vi "Periodic Tasks.vi"(8 "error in":errorcluster) -> ()   [LabVIEW 2014]
doc: "This VI runs in parallel to other tasks. It can contain as many user-defined periodic loops as you need. These can carry out PID or other sorts of timed response."
uses:
  <vilib>/Rock Robotics/WPI/Joystick/WPI_JoystickGetSetRefNum.vi
  <vilib>/Rock Robotics/WPI/RobotDrive/WPI_RobotDriveGetSetRefNum.vi
  Robot Global Data.vi
  <vilib>/Rock Robotics/Network Tables/SD Write Numeric Array.vi
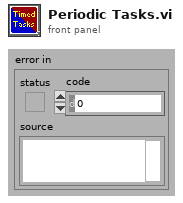
[diagram p1: front panel]
types:
  T1 = typedef "WPI_JoystickDevRef.ctl" = cluster{"Device":T2}
  T2 = typedef "WPI_JoystickDeviceEnum.ctl" = enum16{"USB 0", "USB 1", "USB 2", "USB 3", "USB 4", "USB 5"}
  T3 = typedef "WPI_RobotDriveDevRef.ctl" = cluster{"DevStatus":errorcluster, "Motors[]":T4[], "Square Inputs":bool, "Max Output":dbl}
  T4 = typedef "WPI_MotorControlDeviceRef.ctl" = cluster{"DeviceStatus":errorcluster, "Type":T5, "PWM":cluster{"Controller":T6, "PWM Channel":T7, "DeadBand":T8}, "CAN":cluster{"Device Number":u8, "Control Mode":T9, "Semaphore":T10, "Max Vout":dbl, "TalonSRX Control Mode":T11}, "Invert":bool, "TransformRef":T12, "InvTransformRef":T12}
  T5 = typedef "WPI_MotorControlType.ctl" = enum16{"PWM", "CAN", "CANTalonSRX"}
  T6 = typedef "FPGA_TypedefDigitalModule.ctl" = enum16{"Controller 1"}
  T7 = typedef "FPGA_DIOPWMChannel.ctl" = enum8{"PWM 0", "PWM 1", "PWM 2", "PWM 3", "PWM 4", "PWM 5", "PWM 6", "PWM 7", "PWM 8", "PWM 9", "PWM MXP 0", "PWM MXP 1", "PWM MXP 2", "PWM MXP 3", "PWM MXP 4", "PWM MXP 5", "PWM MXP 6", "PWM MXP 7", "PWM MXP 8", "PWM MXP 9", "Invalid"}
  T8 = typedef "WPI_PWMDeadband.ctl" = cluster{"Name":string, "maxPositivePwm":i32, "minPositivePwm":i32, "centerPwm":i32, "maxNegativePwm":i32, "minNegativePwm":i32, "angularRange":u16}
  T9 = typedef "WPI_CANJaguar_ControlMode.ctl" = enum8{"Percent VBus", "Current", "Speed", "Position", "Voltage"}
  T10 = typedef "Semaphore RefNum" = refnum<k1>
  T11 = typedef "WPI_CANTalonSRX_APIControlMode.ctl" = enum8{"Percent VBus", "Speed", "Position", "Slave", "Unchanged / Invalid"}
  T12 = typedef "WPI_PWMTransform_ConPane.ctl" = refnum<vi>
  T13 = cluster{"JoystickDevRef":T1, "RobotDriveDevRef":T3}
  T14 = typedef "Vector.ctl" = cluster{"Enum":T15, "Data":dbl}
  T15 = typedef "DriveControl.ctl" = enum16{"Drive", "Turn"}
  T16 = typedef "TeleopDriveGroup.ctl" = cluster{"Left/Right":dbl, "Forward/Back":dbl, "Enable Slowdown":bool}
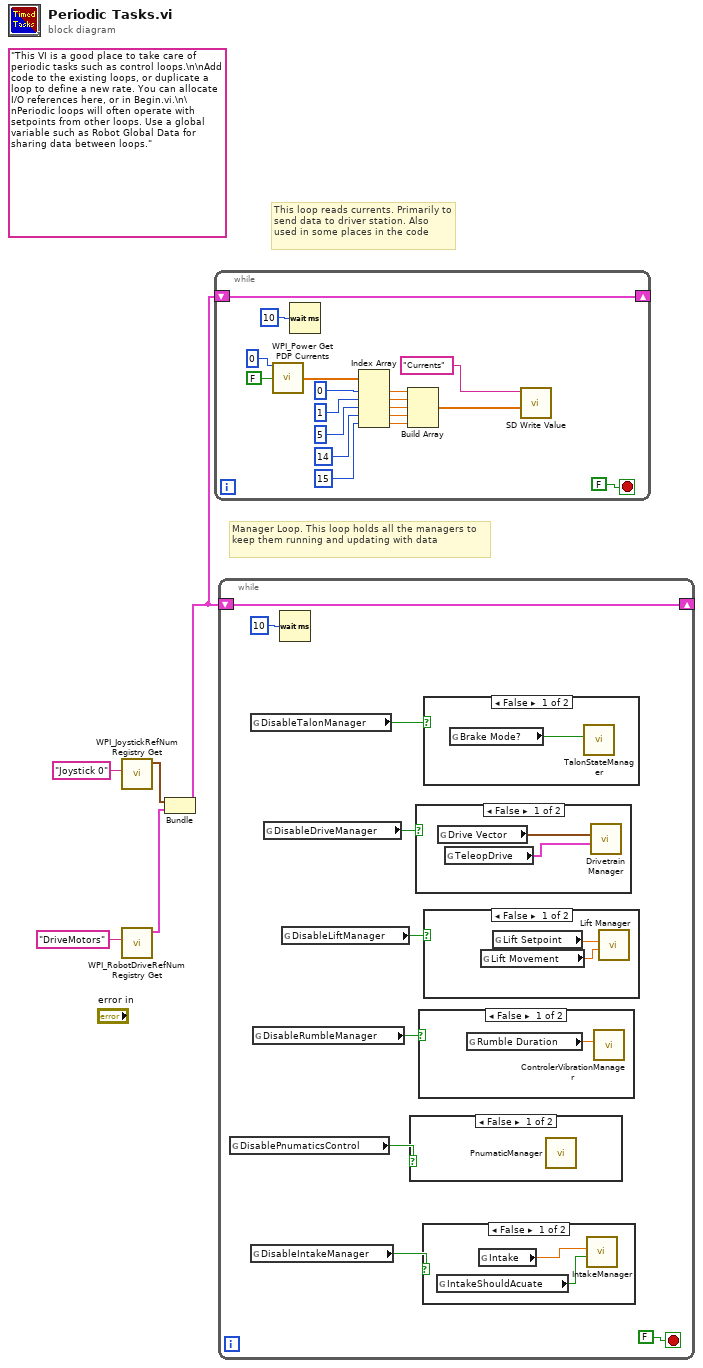
[diagram p0: block diagram]
diagram:
  (unwired) "This VI is a good place to take care of periodic tasks such as control loops.\n\nAdd code to the existing loops, or duplicate a loop to define a new rate. You can allocate I/O references here, or in Begin.vi.\n\nPeriodic loops will often operate with setpoints from other loops. Use a global variable such as Robot Global Data for sharing data between loops."
  # "This loop reads currents. Primarily to send data to driver station. Also used in some places in the code"
  # "Manager Loop. This loop holds all the managers to keep them running and updating with data"
  n1 = call <vilib>:"WPI_JoystickRefNum Registry Get.vi"("refnum name"="Joystick 0") -> ("JoystickDevRef"=w3:T1)  [unwired: 1 in, 9 out]
  n2 = call <vilib>:"WPI_RobotDriveRefNum Registry Get.vi"("refnum name"="DriveMotors") -> ("RobotDriveDevRef"=w2:T3)  [unwired: 1 in, 9 out]
  n3 = Bundle("JoystickDevRef"=w3, "RobotDriveDevRef"=w2) -> (w1:T13)  [unwired: 1 out]
  n4 = while {
    shift-right: [w21] -> _
    shift-left: w1 -> [w21]
    stop <- FALSE stop-if-true
    n5 = call <vilib>:"WPI_Power Get PDP Currents.vi"("Power Distribution Panel (0)"=u8 0, "Tare Currents?"=FALSE) -> ("all currents (A)"=w12:dbl[])  [unwired: 11 in, 2 out]
    n6 = Wait (ms)(milliseconds to wait=u32 10) -> ()  [unwired: 1 out]
    n7 = Index Array(array=w12, index #1=0 ("index"), index #2=1 ("index"), index #3=5 ("index"), index #4=14 ("index"), index #5=15 ("index")) -> (element #1=w7:dbl, element #2=w8:dbl, element #3=w9:dbl, element #4=w10:dbl, element #5=w11:dbl)
    n8 = Build Array(w7, w8, w9, w10, w11) -> (w6:dbl[])
    n9 = call-poly <vilib>:"SD Write Value.vi"("Numeric Array"=w6, "Name"="Currents") -> ()  [unwired: 8 in, 2 out]
  }
  n10 = while {
    shift-right: [w30] -> _
    shift-left: w1 -> [w30]
    stop <- FALSE stop-if-true
    n11 = global read "Robot Global Data.vi" "DisablePnumaticsControl"() -> (w26:bool)
    n12 = global read "Robot Global Data.vi" "DisableTalonManager"() -> (w25:bool)
    n13 = global read "Robot Global Data.vi" "DisableIntakeManager"() -> (w24:bool)
    n14 = global read "Robot Global Data.vi" "DisableRumbleManager"() -> (w27:bool)
    n15 = global read "Robot Global Data.vi" "DisableDriveManager"() -> (w28:bool)
    n16 = Wait (ms)(milliseconds to wait=u32 10) -> ()  [unwired: 1 out]
    n17 = global read "Robot Global Data.vi" "DisableLiftManager"() -> (w29:bool)
    n18 = case shown="False" w26 {
      frame False {
        n19 = call "PnumaticManager.vi"() -> ()  [unwired: 12 in]
      }
      frame True {
      }
    }
    n20 = case shown="False" w28 {
      frame False {
        n21 = global read "Robot Global Data.vi" "Drive Vector"() -> (w38:T14)
        n22 = global read "Robot Global Data.vi" "TeleopDrive"() -> (w37:T16)
        n23 = call "Drivetrain Manager.vi"("DriveDirections"=w37, "Vector"=w38) -> ()  [unwired: 10 in]
      }
      frame True {
      }
    }
    n24 = case shown="False" w27 {
      frame False {
        n25 = global read "Robot Global Data.vi" "Rumble Duration"() -> (w36:dbl)
        n26 = call "ControlerVibrationManager.vi"("Setpoint Duration"=w36) -> ()  [unwired: 11 in]
      }
      frame True {
      }
    }
    n27 = case shown="False" w24 {
      frame False {
        n28 = global read "Robot Global Data.vi" "IntakeShouldAcuate"() -> (w33:bool)
        n29 = global read "Robot Global Data.vi" "Intake"() -> (w34:dbl)
        n30 = call "IntakeManager.vi"("PistonState"=w33, "Intake"=w34) -> ()  [unwired: 10 in]
      }
      frame True {
      }
    }
    n31 = case shown="False" w25 {
      frame False {
        n32 = global read "Robot Global Data.vi" "Brake Mode?"() -> (w35:bool)
        n33 = call "TalonStateManager.vi"("state"=w35) -> ()  [unwired: 11 in]
      }
      frame True {
      }
    }
    n34 = case shown="False" w29 {
      frame False {
        n35 = global read "Robot Global Data.vi" "Lift Movement"() -> (w39:dbl)
        n36 = global read "Robot Global Data.vi" "Lift Setpoint"() -> (w40:dbl)
        n37 = call "Lift Manager.vi"("Manual Lift Setpoint"=w39, "Setpoint"=w40) -> ()  [unwired: 9 in, 1 out]
      }
      frame True {
      }
    }
  }
